vi "test_pid1.vi"() -> ()   [LabVIEW 2013]
panel:
  out "sum":i16
  out "Waveform Graph 4":dbl[](graph)
  out "Waveform Graph 3":dbl[](graph)
  out "Waveform Graph 2":i16[](graph)
  out "Waveform Graph":dbl[](graph)
  out "atan2(y,x)":dbl
  in  "Ki*Tau":fxp<+/-,32,4>=0.010000001639127731
  in  "Kp":fxp<+/-,32,4>=0.10000000149011612
  in  "Kd/Tau":fxp<+/-,32,4>
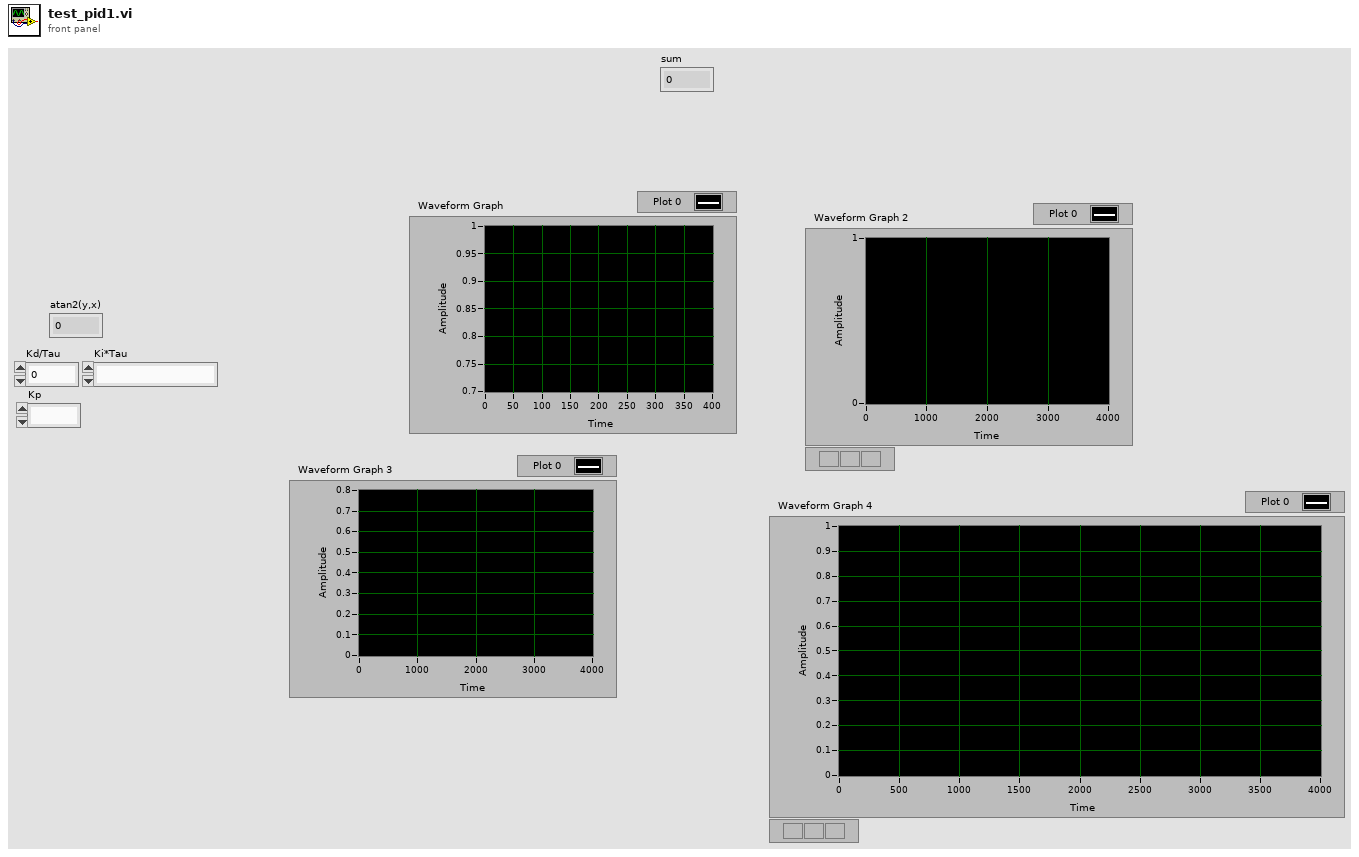
[diagram p1: front panel]
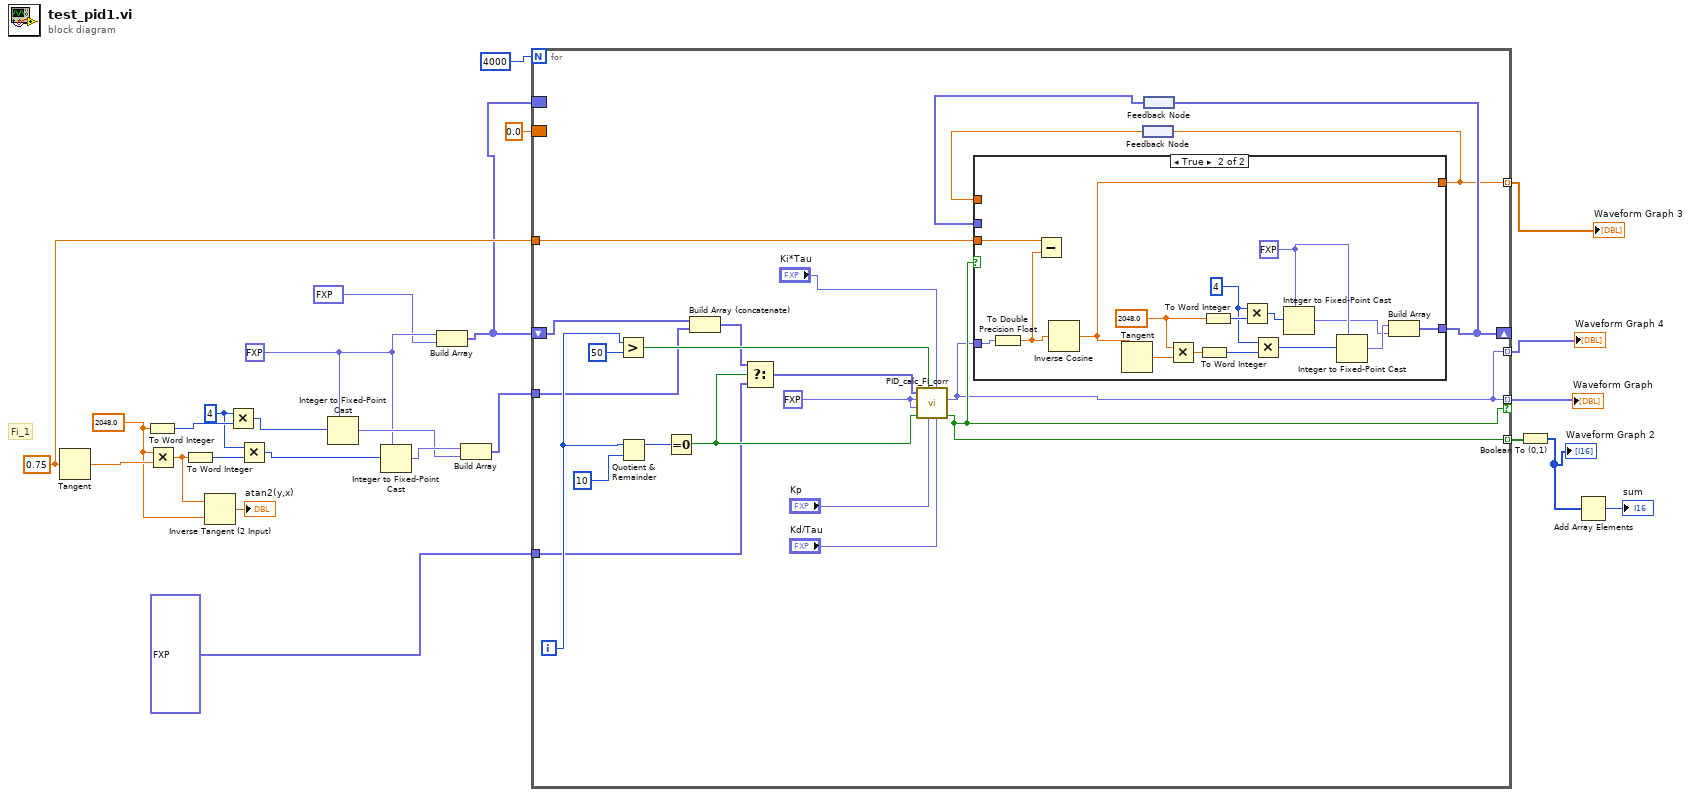
[diagram p0: block diagram]
diagram:
  w13 = i16 4 ("x")
  w9 = fxp<+/-,16,14> 0.0 ("Q in")
  w4 = 0.75 ("x")
  w20 = 2048.0 ("x")
  # "Fi_1"
  n1 = Tangent(1:w4) -> (0:w25:dbl)
  n2 = To Word Integer(number=w20) -> (16bit integer=w16:i16)
  n3 = Multiply(x=w20, y=w25) -> (x*y=w21:dbl)
  n4 = To Word Integer(number=w21) -> (16bit integer=w14:i16)
  n5 = Inverse Tangent (2 Input)(1:w20, 2:w21) -> (0:→"atan2(y,x)":dbl)
  n6 = Multiply(x=w13, y=w16) -> (x*y=w15:i16)
  n7 = Multiply(x=w13, y=w14) -> (x*y=w12:i16)
  n8 = Integer to Fixed-Point Cast(fixed-point type=w9, integer=w15) -> (fixed-point=w17:fxp<+/-,16,14>)
  n9 = Integer to Fixed-Point Cast(fixed-point type=w9, integer=w12) -> (fixed-point=w18:fxp<+/-,16,14>)
  n10 = Build Array(w9, fxp<+/-,16,14> 2048.0 ("element")) -> (w2:fxp<+/-,16,14>[])
  n11 = Build Array(w18, w17) -> (w23:fxp<+/-,16,14>[])
  n12 = for {
    N: 4000 -> [_]
    tunnel: fxp<+/-,16,14>[] [0.0, 0.0, 0.0, 0.0] ("Data in") -> [w39]
    tunnel: w23 -> [w38]
    tunnel: [w27] -> w11 mode=indexing if=w30
    tunnel: [w30] -> w10 mode=indexing
    shift-right: [w37] -> _
    shift-left: w2 -> [w26]
    tunnel: [w35] -> w8 mode=indexing
    border: w2 -> [_]
    tunnel: [w27] -> w7 mode=indexing
    tunnel: w4 -> [w29]
    border: 0.0 -> [_]
    i -> [w44]
    w32 = fxp<+/-,32,4> 0.0 ("Fi_start")
    n13 = Greater?(x=w44, y=50) -> (0:w45:bool)
    n14 = Quotient & Remainder(x=w44, y=10) -> (x-y*floor(x/y)=w42:i32)  [unwired: 1 out]
    n15 = Equal To 0?(x=w42) -> (x = 0?=w41:bool)
    n16 = Build Array (concatenate)(w26, w38) -> (w28:fxp<+/-,16,14>[])
    n17 = Select(t=w28, s=w41, f=w39) -> (s? t:f=w40:fxp<+/-,16,14>[])
    n18 = call "PID_calc_Fi_corr.vi"("Kd/Tau"="Kd/Tau", "Ki*Tau"="Ki*Tau", "Kp"="Kp", "Enabled"=w45, "input valid"=w41, "Fi_delta"=w32, "Fi_start"=w32, "Data in"=w40) -> ("output valid"=w30:bool, "cos_fi_korr"=w27:fxp<+/-,16,2>)  [unwired: 1 in, 1 out]
    n19 = feedback #1() -> (w34:dbl)
    n20 = feedback #2() -> (w36:fxp<+/-,16,14>[])
    n21 = case shown="True" w30 {
      tunnel: w27 -> [_ w65]
      tunnel: [w49 w55] -> w37
      tunnel: [w48 w50] -> w35
      tunnel: w36 -> [w49 _]
      tunnel: w34 -> [w48 _]
      tunnel: w29 -> [_ w52]
      frame False {
      }
      frame True {
        w57 = i16 4 ("x")
        w63 = fxp<+/-,16,14> 0.0 ("Q in")
        w61 = 2048.0 ("x")
        n22 = To Double Precision Float(number=w65) -> (double precision float=w51:dbl)
        n23 = Subtract(x=w52, y=w51) -> ()  [unwired: 1 out]
        n24 = Inverse Cosine(1:w51) -> (0:w50:dbl)
        n25 = Tangent(1:w50) -> (0:w64:dbl)
        n26 = Multiply(x=w61, y=w64) -> (x*y=w62:dbl)
        n27 = To Word Integer(number=w62) -> (16bit integer=w58:i16)
        n28 = To Word Integer(number=w61) -> (16bit integer=w60:i16)
        n29 = Multiply(x=w57, y=w60) -> (x*y=w59:i16)
        n30 = Multiply(x=w57, y=w58) -> (x*y=w56:i16)
        n31 = Integer to Fixed-Point Cast(fixed-point type=w63, integer=w59) -> (fixed-point=w53:fxp<+/-,16,14>)
        n32 = Integer to Fixed-Point Cast(fixed-point type=w63, integer=w56) -> (fixed-point=w54:fxp<+/-,16,14>)
        n33 = Build Array(w54, w53) -> (w55:fxp<+/-,16,14>[])
      }
    }
    n34 = feedback-in #1(w35) -> ()
    n35 = feedback-in #2(w37) -> ()
  }
  "Waveform Graph" <- w11
  "Waveform Graph 3" <- w8
  "Waveform Graph 4" <- w7
  n36 = Boolean To (0,1)(Boolean=w10) -> (0, 1=w6:i16[])
  "Waveform Graph 2" <- w6
  n37 = Add Array Elements(numeric array=w6) -> (sum=→"sum":i16)
